vi "ZMC Step Run.vi"(5 "iLineNum":u32, 6 "ifilenum":u8, 7 "bifBreakAll":u8, 8 "error in (no error)":errorcluster caption="错误输入（无错误）", 9 "Stepmode":u8, 10 "taskid":u16, 11 "handle":u32) -> (0 "error out":errorcluster caption="错误输出", 2 "function return":i32, 3 "handle out":u32)   [LabVIEW 2015, in "zauxdll.lvlib"]
doc: "int32 __stdcall ZMC_StepRun(ZMC_HANDLE handle, uint16 taskid, uint8 Stepmode, uint8 bifBreakAll, uint8 ifilenum, uint32 iLineNum);"
uses:
  zauxdll.lvlib
  zmotion.dll
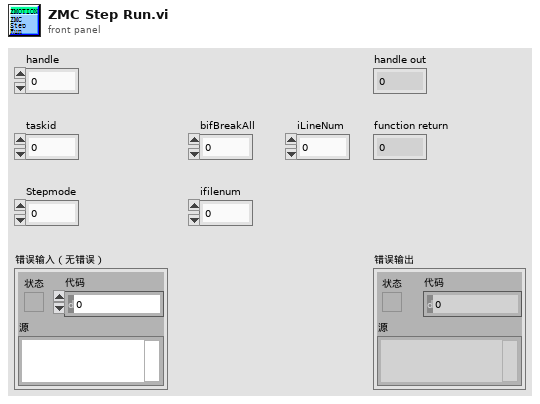
[diagram p1: front panel]
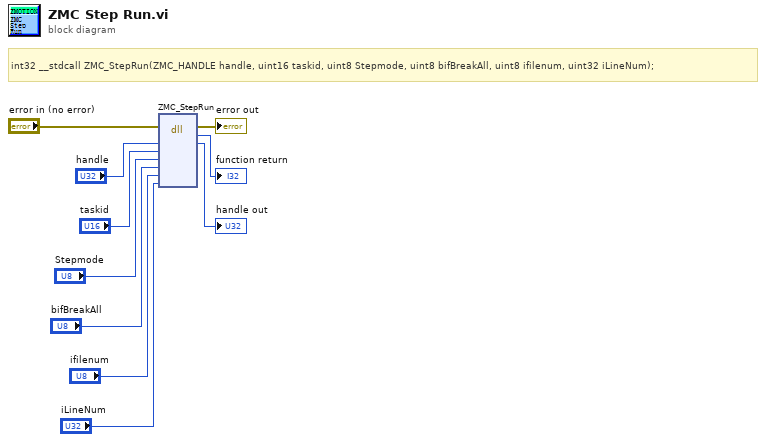
[diagram p0: block diagram]
diagram:
  # "int32 __stdcall ZMC_StepRun(ZMC_HANDLE handle, uint16 taskid, uint8 Stepmode, uint8 bifBreakAll, uint8 ifilenum, uint32 iLineNum);"
  n1 = dll-call lib="C:/Users/VIC/Desktop/GOGORO_SA/system/LLB/zmotion/zaux/zmotion.*" fn="ZMC_StepRun"(error in="error in (no error)", "handle"="handle", "taskid"="taskid", "Stepmode"="Stepmode", "bifBreakAll"="bifBreakAll", "ifilenum"="ifilenum", "iLineNum"="iLineNum") -> (error out=→"error out":errorcluster, →"function return":i32, "handle"=→"handle out":u32)  [unwired: 7 in, 1 out]
